vi "RT Driver VI.vi"(7 "Operation":T1, 11 "Device Reference in":T2 format="%.0x") -> (0 "Error Code":i32)   [LabVIEW 2019, in "Fuel Injector Analysis Addon Engine.lvlib"]
uses:
  Fuel Injector Analysis Addon Engine.lvlib
  <vilib>/rvi/interface/nirviCloseFPGA/nirviCloseFPGA.xnode
  <vilib>/NI/NIVS Inline Async API/_VS Inline Async API/VS Inline Async API/VS Inline Async API.lvclass
  <vilib>/rvi/interface/nirviMethod/nirviMethod.xnode
  <vilib>/rvi/interface/nirviMethod/StockFPGA_InlinedMethodWaitForSingleIRQ.vi
  <vilib>/FPGAPlugInAG/Dynamic/niLvFpga_WaitOnIrq_Dynamic.vi
  <vilib>/FPGAPlugInAG/Dynamic/niLvFpga_AcknowledgeIrq_Dynamic.vi
  <vilib>/NI VeriStand/Custom Device API/Custom Device API.lvlib
  <vilib>/FPGAPlugInAG/Dynamic/niLvFpga_Close_Dynamic.vi
  <vilib>/NI VeriStand/Custom Device API/Get Item Property (Variant).vi
  Addon Shared/Constants.vi
  Addon Shared/Fuel Injector Analysis Addon Shared.lvlib
  Addon Shared/Types/FPGA Data Types.ctl
  Addon Shared/Types/Register.Info.ctl
  Addon Shared/Types/VS.Register.Info.ctl
  <vilib>/NI VeriStand/Custom Device API/Data Reference.ctl
  <vilib>/NI VeriStand/Custom Device API/Block Data Reference.ctl
  <vilib>/NI VeriStand/Custom Device API/Waveform Data Reference.ctl
  Addon Shared/Types/Injector info.ctl
  Addon Shared/Types/Compiled.Settings.ctl
  Addon Shared/Types/Analysis.Channels.Select.ctl
  Addon Shared/Types/Stage.Transition.Types.ctl
  Addon Shared/Types/Stage.PullIn.Types.ctl
  Addon Shared/Types/Stage.Parameters.ctl
  Addon Shared/Types/Shot.Parameters.ctl
  Addon Shared/Types/Compiled.Group.Timing.ctl
  Addon Shared/Types/Compiled.Group.WaveformRefs.ctl
  <vilib>/NI/NIVS Inline Async API/_VS Inline Async API/VS Inline Async API/Types/Error Handling Settings.ctl
  <vilib>/NI/NIVS Inline Async API/_Data Access Engine/Access Type Classes/Write/Write.lvclass
  <vilib>/NI/NIVS Inline Async API/_Data Access Engine/Access Type Classes/Read/Read.lvclass
  <vilib>/NI VeriStand/Custom Device Waveform API/Single Waveform Write (DBL)/Single Waveform Write (DBL).lvclass
  <vilib>/NI VeriStand/Custom Device API/Custom Device Item Ref.ctl
  <vilib>/NI VeriStand/Custom Device API/Hardware Interface Driver VI Operation.ctl
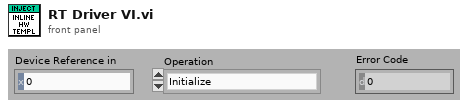
[diagram p1: front panel]
types:
  T1 = typedef "Custom Device API.lvlib/Hardware Interface Driver VI Operation.ctl" = enum16{"Initialize", "Start", "Read Data from HW", "Write Data to HW", "Close"}
  T2 = typedef "Custom Device API.lvlib/Custom Device Item Ref.ctl" = u64
  T3 = typedef "Fuel Injector Analysis Addon Engine.lvlib/Inline State Data.ctl" = cluster{"Name":string, "FPGA Ref":refnum<k20>, "Inline Error":errorcluster, "Async":refnum<class "VS Inline Async API.lvclass">, "FPGA.Registers":T4[], "VS.Registers":T6[], "VS.Registers.Values":dbl[], "# of Registers":u32, "Group.Rate":u32[]}
  T4 = typedef "Fuel Injector Analysis Addon Engine.lvlib/FPGA Refs.ctl" = cluster{"Data Type":T5, "Index":i32, "Length":i32, "Group":i32, "Injector.Core.Setting":refnum<k20>, "Injector.Global.Setting":refnum<k20>, "Injector.MUX.Setting":refnum<k20>, "Injector.Timing":refnum<k20>}
  T5 = typedef "Fuel Injector Analysis Addon Shared.lvlib/FPGA Data Types.ctl" = enum8{"<Null>", "Injector.Core.Setting", "Injector.Global.Setting", "Injector.Mux.Setting", "Injector.Timing"}
  T6 = typedef "Custom Device API.lvlib/Block Data Reference.ctl" = cluster{"Data Reference":T7, "Offset":u64, "Length":u64}
  T7 = typedef "Custom Device API.lvlib/Data Reference.ctl" = i32
  T8 = typedef "VS Inline Async API.lvlib/VS Inline Async API.lvclass/Error Handling Settings.ctl" = cluster{"Write to SystemLog (F)":bool}
  T9 = typedef "Fuel Injector Analysis Addon Shared.lvlib/Compiled.Settings.ctl" = cluster{"Name":string, "RIO.Address":string, "Bitfile.Path":path, "Injectors.Count":u32, "Injectors.Settings":T10[], "Waveform.Refs":T11[], "VS.Registers":cluster{"Block Data refs":T6[], "Values":dbl[]}, "Registers":T13[], "Timing.Registers":T15[], "Mux.Register":T14, "Groups.Settings":T16[]}
  T10 = typedef "Fuel Injector Analysis Addon Shared.lvlib/Injector info.ctl" = cluster{"Results Index":i32, "Waveform Index":i32, "Group":u16}
  T11 = typedef "Fuel Injector Analysis Addon Shared.lvlib/Compiled.Group.WaveformRefs.ctl" = cluster{"WaveformRefs":T12[], "Group":i32}
  T12 = typedef "Custom Device API.lvlib/Waveform Data Reference.ctl" = i32
  T13 = typedef "Fuel Injector Analysis Addon Shared.lvlib/VS.Register.Info.ctl" = cluster{"Index":i32, "Length":i32, "Group":i32, "Register":T14}
  T14 = typedef "Fuel Injector Analysis Addon Shared.lvlib/Register.Info.ctl" = cluster{"Name":string, "Data Type":T5, "Default Value":variant}
  T15 = typedef "Fuel Injector Analysis Addon Shared.lvlib/Compiled.Group.Timing.ctl" = cluster{"Name":string, "Sample rate (S/s)":u32}
  T16 = typedef "Fuel Injector Analysis Addon Shared.lvlib/Shot.Parameters.ctl" = cluster{"Shots":u32, "Shot.InitialVoltage":dbl, "Shot.Stages":u32, "Stages":T17[], "Timeout":dbl, "Results.Count":i32, "Active Edge":bool, "Rate.Hz":u32, "Channels":u32}
  T17 = typedef "Fuel Injector Analysis Addon Shared.lvlib/Stage.Parameters.ctl" = cluster{"Stage.Dwell.Level":dbl, "PullIn.Type":T18, "PullIn.Level":dbl, "Transition.Type":T19, "Transition.Level":dbl, "Results":T20}
  T18 = typedef "Fuel Injector Analysis Addon Shared.lvlib/Stage.PullIn.Types.ctl" = enum8{"Pull In Transition Pulses", "Pull In Transition Current Drop"}
  T19 = typedef "Fuel Injector Analysis Addon Shared.lvlib/Stage.Transition.Types.ctl" = enum8{"Stage Transition Inactive Time", "Stage Transition Voltage Increase", "Stage Transition Current Decrease", "Stage Transition Active Time"}
  T20 = typedef "Fuel Injector Analysis Addon Shared.lvlib/Analysis.Channels.Select.ctl" = cluster{"Pull In Time":bool, "Pull In Max Current":bool, "Pull In Max Voltage":bool, "Pull In Min Voltage":bool, "Pull In Avg Voltage":bool, "Hold Time":bool, "Hold Max Current":bool, "Hold Min Current":bool, "Hold Avg Current":bool, "Hold Max Voltage":bool, "Hold Min Voltage":bool, "Hold Avg Max Voltage":bool, "Hold Avg Min Voltage":bool, "Off Time":bool, "Off Max Current":bool, "Off Min Current":bool, "Off Avg Current":bool, "Off Max Voltage":bool, "Off Min Voltage":bool, "Off Avg Voltage":bool, "Total Voltage Pulses":bool, "Total Stage Time":bool}
  T21 = typedef "Fuel Injector Analysis Addon Engine.lvlib/Async Parameters.ctl" = cluster{"Name":string, "Injectors.Count":u8, "Groups.Settings":T16[], "Groups.InitResults":cluster{"Values":dbl[]}[], "Injectors.Settings":T10[], "Injectors.State":T22[], "DMA.Ref":refnum<k20>, "FPGA.Status":T23, "Search.Data":T24, "Results.Data":T23, "Waveform.Enable":T24, "Waveform.Refs":T11[], "Waveform.Sessions":refnum<class "Single Waveform Write (DBL).lvclass">[]}
  T22 = typedef "Fuel Injector Analysis Addon Engine.lvlib/Injector.State.ctl" = cluster{"Timer":u32, "Events":u64}
  T23 = typedef "Data Access Engine.lvlib/Data Access Engine.lvclass/Write.DVR.ctl" = refnum<data-value>
  T24 = typedef "Data Access Engine.lvlib/Data Access Engine.lvclass/Read.DVR.ctl" = refnum<data-value>
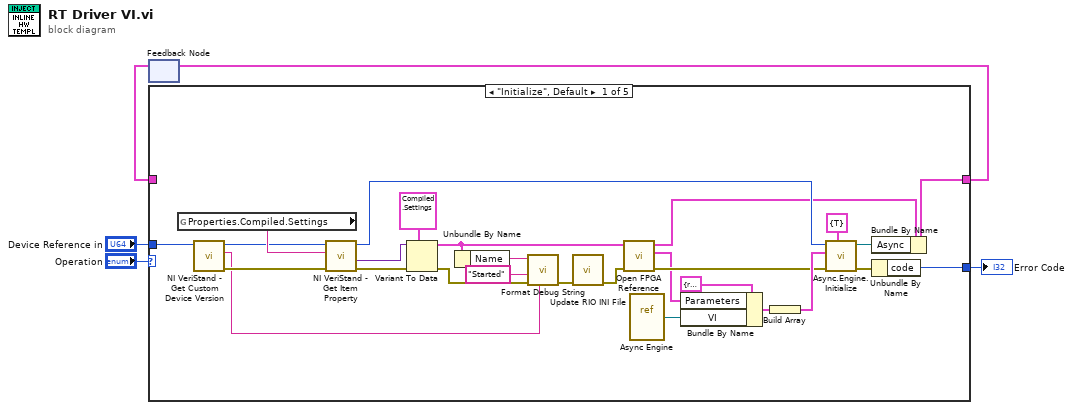
[diagram p0: block diagram]
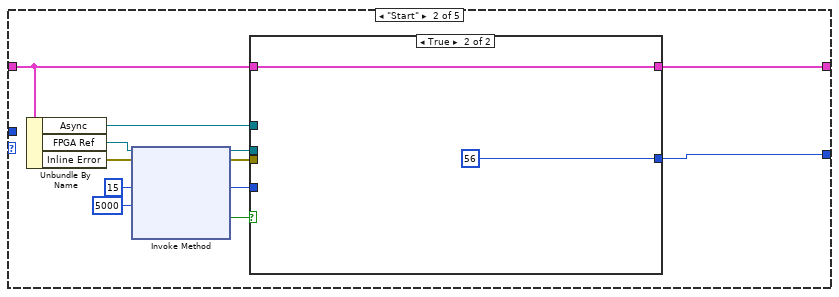
[diagram p2: hidden frame]
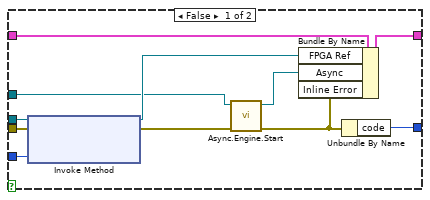
[diagram p3: hidden frame]
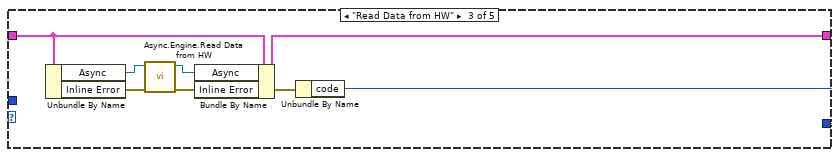
[diagram p4: hidden frame]
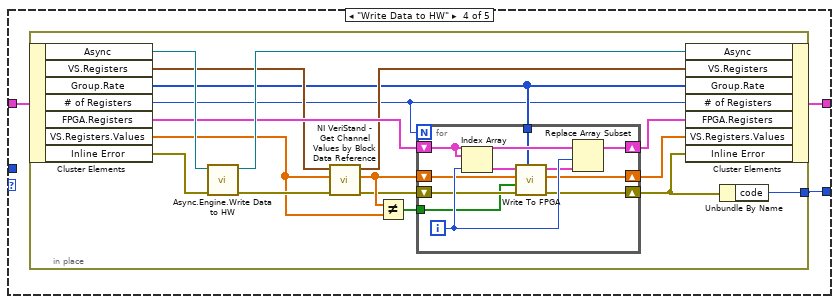
[diagram p5: hidden frame]
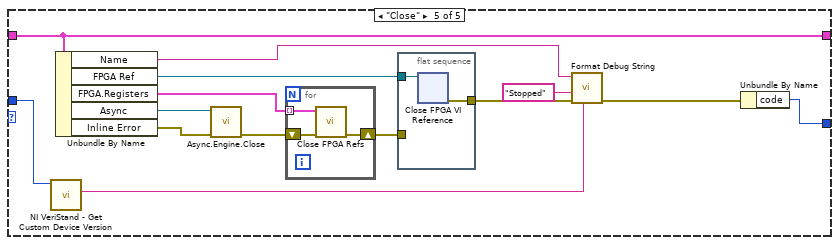
[diagram p6: hidden frame]
diagram:
  n1 = feedback #1() -> (w4:T3)  [unwired: 1 out]
  n2 = case shown="\"Initialize\", Default" "Operation" {
    tunnel: w4 -> [_ w35 w63 w66 w107]
    tunnel: "Device Reference in" -> [w16 _ _ _ w100]
    tunnel: [w32 w33 w61 w64 w102] -> w2
    tunnel: [w31 w34 w62 w65 w107] -> w1
    frame "Initialize", Default {
      n3 = global read "Constants.vi" "Properties.Compiled.Settings"() -> (w25:string)
      n4 = call <vilib>:"NI VeriStand - Get Custom Device Version.vi"("Device Ref in"=w16) -> ("error out"=w14:errorcluster, "Value"=w9:string, "Device Ref out"=w15:T2)  [unwired: 8 in]
      n5 = call-poly <vilib>:"NI VeriStand - Get Item Property.vi"("error in (no error)"=w14, "Property Name"=w25, "Item Ref in"=w15) -> ("error out"=w24:errorcluster, "Value"=w23:variant, "Item Ref out"=w21:T2)  [unwired: 5 in, 1 out]
      n6 = Variant To Data(error in=w24, type=T9 {"Name"="", "RIO.Address"="", "Bitfile.Path"=path "", "Injectors.Count"=0, "Injectors.Settings"=[], "Waveform.Refs"=[], "VS.Registers"={"Block Data refs"=[], "Values"=[]}, "Registers"=[], "Timing.Registers"=[], "Mux.Register"={"Name"="", "Data Type"=enum."<Null>", "Default Value"=variant(dbl 0.0)}, "Groups.Settings"=[]} ("Settings.Compiled"), Variant=w23) -> (data=w8:T9, error out=w11:errorcluster)
      n7 = Unbundle By Name(w8) -> ("Name"=w7:string)
      n8 = call "Format Debug String.vi"("Version"=w9, "error in (no error)"=w11, "State"="Started", "Name"=w7) -> ("error out"=w10:errorcluster)  [unwired: 7 in]
      n9 = call "Update RIO INI File.vi"("error in (no error)"=w10) -> ("error out"=w17:errorcluster)  [unwired: 10 in]
      n10 = call "Open FPGA Reference.vi"("Error In"=w17, "Settings.Compiled"=w8) -> ("Error Out"=w20:errorcluster, "Async Parameters"=w18:T21, "Inline State Data out"=w19:T3)  [unwired: 7 in]
      n11 = vi-ref "Async Engine.vi"() -> (w13:refnum<vi>)
      n12 = Bundle By Name(cluster=cluster{"VI":refnum<vi>, "Parameters":variant} {"VI"=refnum, "Parameters"=variant} ("Process"), "Parameters"=w18, "VI"=w13) -> (w29:cluster{"VI":refnum<vi>, "Parameters":variant})
      n13 = Build Array(w29) -> (w28:cluster{"VI":refnum<vi>, "Parameters":variant}[])
      n14 = call <vilib>:"Async.Engine.Initialize.vi"("Error Log Settings"=T8 {"Write to SystemLog (F)"=TRUE}, "error in (no error)"=w20, "Processes"=w28, "Custom Device Ref"=w21) -> ("error out"=w27:errorcluster, "Async"=w26:refnum<class "VS Inline Async API.lvclass">)  [unwired: 6 in]
      n15 = Bundle By Name(cluster=w19, "Async"=w26) -> (w31:T3)
      n16 = Unbundle By Name(w27) -> ("code"=w32:i32)
    }
    frame "Start" {
      w41 = 15 ("IRQ Number(s)")
      n17 = Unbundle By Name(w35) -> ("Async"=w36:refnum<class "VS Inline Async API.lvclass">, "FPGA Ref"=w37:refnum<k20>, "Inline Error"=w38:errorcluster)
      n18 = xnode "Invoke Method"("FPGA VI Reference In"=w37, "error in"=w38, "IRQ Number(s)"=w41, "Timeout (ms)"=5000) -> ("FPGA VI Reference Out"=w39:refnum<k20>, "error out"=w40:errorcluster, "Timed Out"=w43:bool)  [unwired: 1 out]
      n19 = case shown="True" w43 {
        tunnel: [w54 56 ("code")] -> w33
        tunnel: w35 -> [w53 w55]
        tunnel: [w52 w55] -> w34
        tunnel: w39 -> [w51 _]
        tunnel: w40 -> [w50 _]
        tunnel: w41 -> [w49 _]
        tunnel: w36 -> [w46 _]
        frame False {
          n20 = xnode "Invoke Method"("FPGA VI Reference In"=w51, "error in"=w50, "IRQ Number(s)"=w49) -> ("FPGA VI Reference Out"=w48:refnum<k20>, "error out"=w44:errorcluster)
          n21 = call <vilib>:"Async.Engine.Start.vi"("error in (no error)"=w44, "VS Inline Async API in"=w46) -> ("error out"=w47:errorcluster, "VS Inline Async API out"=w45:refnum<class "VS Inline Async API.lvclass">)  [unwired: 8 in]
          n22 = Bundle By Name(cluster=w53, "FPGA Ref"=w48, "Async"=w45, "Inline Error"=w47) -> (w52:T3)
          n23 = Unbundle By Name(w47) -> ("code"=w54:i32)
        }
        frame True {
        }
      }
    }
    frame "Read Data from HW" {
      n24 = Unbundle By Name(w63) -> ("Async"=w59:refnum<class "VS Inline Async API.lvclass">, "Inline Error"=w60:errorcluster)
      n25 = call <vilib>:"Async.Engine.Read Data from HW.vi"("error in"=w60, "Async in"=w59) -> ("error out"=w57:errorcluster, "Async out"=w58:refnum<class "VS Inline Async API.lvclass">)  [unwired: 8 in]
      n26 = Bundle By Name(cluster=w63, "Async"=w58, "Inline Error"=w57) -> (w62:T3)
      n27 = Unbundle By Name(w57) -> ("code"=w61:i32)
    }
    frame "Write Data to HW" {
      n28 = in-place {
        in-place-border: [w67] -> w64
        n29 = in-place-cluster #2(w66) -> ("Async"=w79:refnum<class "VS Inline Async API.lvclass">, "VS.Registers"=w72:T6[], "Group.Rate"=w70:u32[], "# of Registers"=w69:u32, "FPGA.Registers"=w76:T4[], "VS.Registers.Values"=w73:dbl[], "Inline Error"=w78:errorcluster)
        n30 = call <vilib>:"Async.Engine.Write Data to HW.vi"("error in (no error)"=w78, "VS Inline Async API in"=w79) -> ("error out"=w80:errorcluster, "VS Inline Async API out"=w77:refnum<class "VS Inline Async API.lvclass">)  [unwired: 8 in]
        n31 = call <vilib>:"NI VeriStand - Get Channel Values by Block Data Reference.vi"("error in (no error)"=w80, "Values Array in"=w73, "Block Data Ref"=w72) -> ("error out"=w81:errorcluster, "Values Array out"=w82:dbl[], "Block Data Ref dup"=w71:T6[])  [unwired: 6 in]
        n32 = Not Equal?(x=w82, y=w73) -> (x != y?=w83:bool[])
        n33 = for {
          N: w69 -> [_]
          shift-right: [w87] -> w74
          shift-left: w82 -> [w88]
          shift-right: [w94] -> w75
          shift-left: w76 -> [w93]
          shift-right: [w90] -> w68
          shift-left: w81 -> [w91]
          tunnel: w83 -> [w89]
          tunnel: w70 -> [w84]
          i -> [w92]
          n34 = Index Array(array=w93, index=w92) -> (element=w86:T4)
          n35 = call "Write To FPGA.vi"("Group.Rate"=w84, "error in (no error)"=w91, "Changed?"=w89, "Values"=w88, "FPGA Refs"=w86) -> ("error out"=w90:errorcluster, "Values out"=w87:dbl[], "FPGA Refs"=w85:T4)  [unwired: 4 in]
          n36 = Replace Array Subset(array=w93, new element=w85, index=w92) -> (w94:T4[])
        }
        n37 = in-place-cluster #2("Async"=w77, "VS.Registers"=w71, "Group.Rate"=w70, "# of Registers"=w69, "FPGA.Registers"=w75, "VS.Registers.Values"=w74, "Inline Error"=w68) -> (w65:T3)
        n38 = Unbundle By Name(w68) -> ("code"=w67:i32)
      }
    }
    frame "Close" {
      n39 = call <vilib>:"NI VeriStand - Get Custom Device Version.vi"("Device Ref in"=w100) -> ("Value"=w96:string)  [unwired: 8 in, 2 out]
      n40 = Unbundle By Name(w107) -> ("Name"=w95:string, "FPGA Ref"=w108:refnum<k20>, "FPGA.Registers"=w103:T4[], "Async"=w105:refnum<class "VS Inline Async API.lvclass">, "Inline Error"=w106:errorcluster)
      n41 = call <vilib>:"Async.Engine.Close.vi"("error in (no error)"=w106, "Async in"=w105) -> ("error out"=w104:errorcluster)  [unwired: 8 in, 1 out]
      n42 = for {
        shift-right: [w112] -> w101
        shift-left: w104 -> [w113]
        tunnel: w103 -> [w111] mode=indexing
        n43 = call "Close FPGA Refs.vi"("error in (no error)"=w113, "FPGA Refs"=w111) -> ("error out"=w112:errorcluster)  [unwired: 9 in]
      }
      n44 = flat-sequence {
        tunnel: w108 -> [w110]
        tunnel: w101 -> [_]
        tunnel: [w109] -> w98
        frame #0 {
          n45 = xnode "Close FPGA VI Reference"("FPGA VI Reference In"=w110) -> ("error out"=w109:errorcluster)  [unwired: 1 in]
        }
      }
      n46 = call "Format Debug String.vi"("Version"=w96, "error in (no error)"=w98, "State"="Stopped", "Name"=w95) -> ("error out"=w97:errorcluster)  [unwired: 7 in]
      n47 = Unbundle By Name(w97) -> ("code"=w102:i32)
    }
  }
  "Error Code" <- w2
  n48 = feedback-in #1(w1) -> ()
